vi "Read Sender.vi"(11 "Finish Msg in":refnum<class "Finish Msg.lvclass">) -> (2 "Sender":refnum<class "Sender.lvclass">)   [LabVIEW 2025, in "jettl.lvlib" / "Finish Msg.lvlib" / "Finish Msg.lvclass"]
uses:
  Finish Msg.lvclass
  Sender/Sender/Sender.lvclass
  Finish Msg.lvclass/Finish Msg.ctl
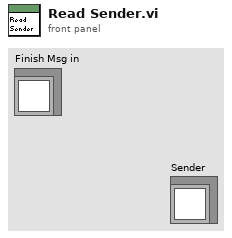
[diagram p1: front panel]
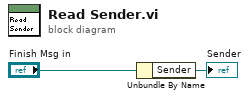
[diagram p0: block diagram]
diagram:
  n1 = Unbundle By Name("Finish Msg in") -> ("Sender"=→"Sender":refnum<class "Sender.lvclass">)
